vi "coag_dose_to_flow.vi"(4 "State":i16, 5 "Time":dbl format="%.2f", 6 "Sensor Values":dbl[](array[numeric]), 7 "Set Points":dbl[](array[numeric])) -> (0 "required data":T1={"Set Point names"=["coagulant dose (mg/L)", "manual flow (mL/s)", ""], "required number of setpoints"=2, "required number of sensors"=1, "Sensor names"=["raw flow rate (L/s)"]}, 3 "output value":dbl)   [LabVIEW 2019]
uses:
  Global Plantita Parameters.vi
panel:
  # "Enter the correct information for this control code in the required data structure below. Then make the current value default by right clicking on the border of the data structure. Select \"data operations\" and then select \"make current value default\". These values will be displayed by process controller."
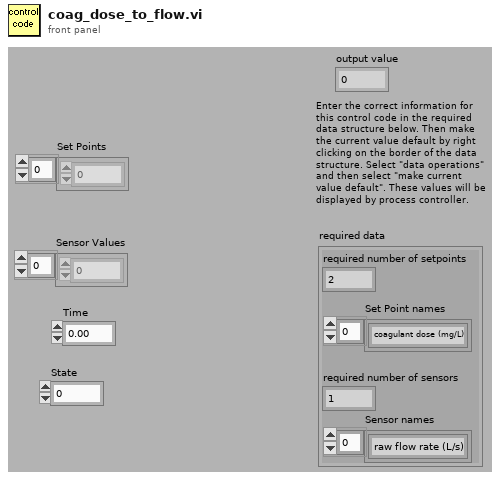
[diagram p1: front panel]
types:
  T1 = cluster{"Set Point names":string[], "required number of setpoints":u8, "required number of sensors":u8, "Sensor names":string[]}
  T2 = cluster{"height_ff (m)":dbl, "C_coag_stock (g/L)":dbl, "flocculation_time(min)":dbl, "clarification_time(min)":dbl, "data_interval (min)":dbl}
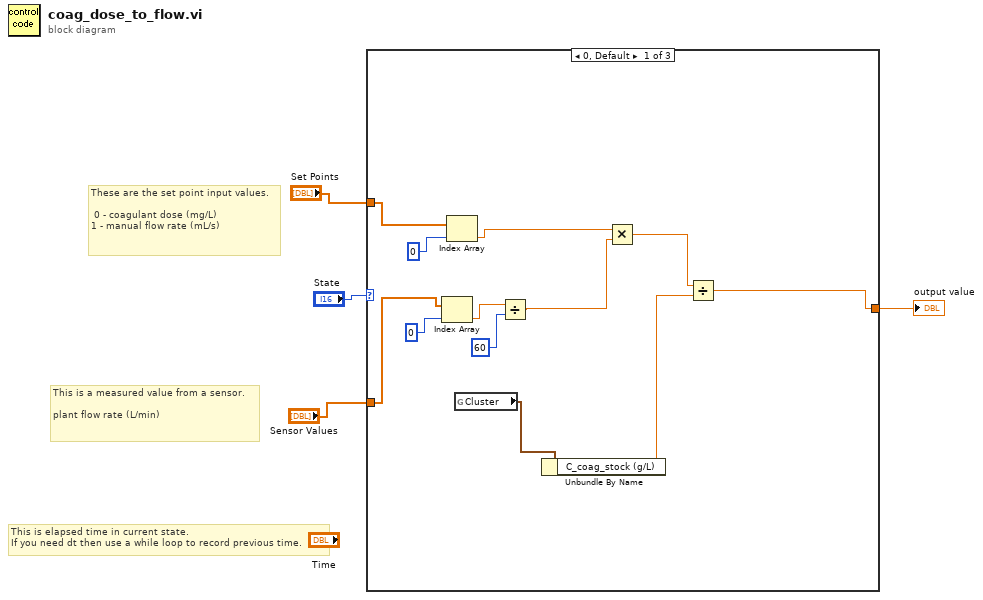
[diagram p0: block diagram]
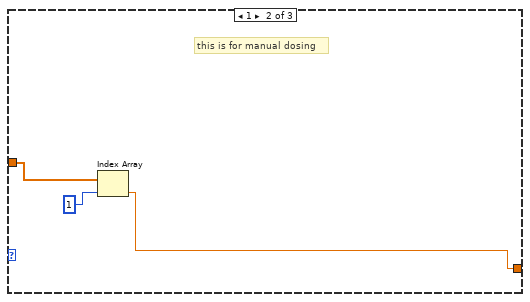
[diagram p2: hidden frame]
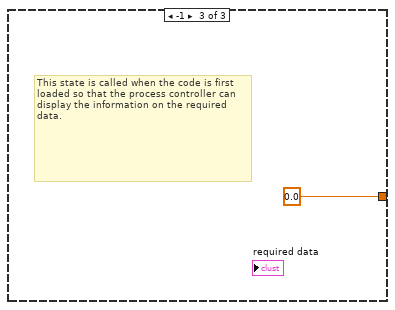
[diagram p3: hidden frame]
diagram:
  # "These are the set point input values.\n\n 0 - coagulant dose (mg/L)\n1 - manual flow rate (mL/s)"
  # "This is a measured value from a sensor.\n\nplant flow rate (L/min)"
  # "This is elapsed time in current state.\nIf you need dt then use a while loop to record previous time."
  n1 = case shown="0, Default" "State" {
    tunnel: [w15 w17 0.0 ("fraction on")] -> w1
    tunnel: "Set Points" -> [w13 w18 _]
    tunnel: "Sensor Values" -> [w11 _ _]
    frame 0, Default {
      n2 = Index Array(array=w11, index=0) -> (element=w7:dbl)
      n3 = Index Array(array=w13, index=0) -> (element=w12:dbl)
      n4 = global read "Global Plantita Parameters.vi" "Cluster"() -> (w9:T2)
      n5 = Divide(x=w7, y=60) -> (x/y=w6:dbl)
      n6 = Unbundle By Name(w9) -> ("C_coag_stock (g/L)"=w8:dbl)
      n7 = Multiply(x=w12, y=w6) -> (x*y=w16:dbl)
      n8 = Divide(x=w16, y=w8) -> (x/y=w15:dbl)
    }
    frame 1 {
      # "this is for manual dosing"
      n9 = Index Array(array=w18, index=1) -> (element=w17:dbl)
    }
    frame -1 {
      # "This state is called when the code is first loaded so that the process controller can display the information on the required data."
    }
  }
  "output value" <- w1
